vi "Write Homed Status.vi"(8 "error in (no error)":errorcluster, 10 "Homed?":bool, 11 "Axis in":refnum<class "Axis.lvclass">) -> (0 "error out":errorcluster, 3 "Axis out":refnum<class "Axis.lvclass">)   [LabVIEW 2018, in "Axis.lvlib" / "Axis.lvclass"]
uses:
  Axis.lvclass
  Axis.lvclass/Axis.ctl
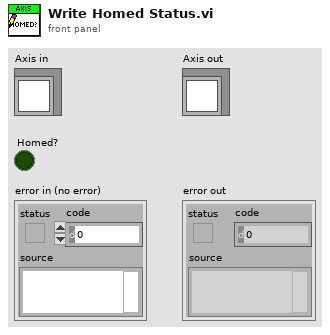
[diagram p1: front panel]
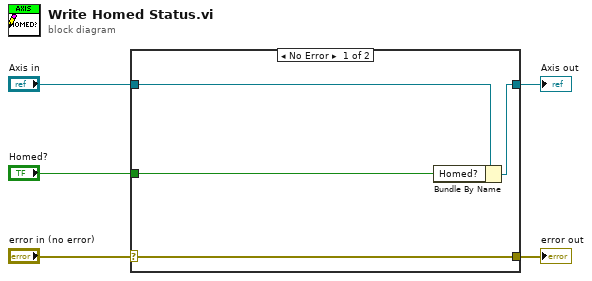
[diagram p0: block diagram]
diagram:
  n1 = case shown="No Error" "error in (no error)" {
    selector: "error in (no error)" -> [w9 w10]
    tunnel: [w9 w10] -> w4
    tunnel: [w7 w11] -> w2
    tunnel: "Axis in" -> [w8 w11]
    tunnel: "Homed?" -> [w6 _]
    frame No Error {
      n2 = Bundle By Name(cluster=w8, "Homed?"=w6) -> (w7:refnum<class "Axis.lvclass">)
    }
    frame Error {
    }
  }
  "error out" <- w4
  "Axis out" <- w2
